vi "Set Start Parameter.vi"(8 "error in (no error)":errorcluster, 10 "Start Parameter":T2={"Windows Titel"="", "Start WorkDir"=path "C:/Users/user/Desktop/test/WorkDir", "Camera ConfigDir"=path "C:/Users/user/Desktop/test/ConfigDir", "Camera"="TestCam"}, 11 "HIJ 4 Aligment Cams Launcher in":refnum<class "HIJ 3 Aligment Cams Launcher.lvclass">) -> (0 "error out":errorcluster, 3 "HIJ 4 Aligment Cams Launcher out":refnum<class "HIJ 3 Aligment Cams Launcher.lvclass">)   [LabVIEW 2014, in "HIJ 3 Alignment Cams App.lvlib" / "HIJ 3 Aligment Cams Launcher.lvclass"]
uses:
  HIJ 3 Aligment Cams Launcher.lvclass
  <vilib>/userdefined/High Color/IMAQdx.ctl
  HIJ 3 Alignment Cams App/HIJ 3 Alignment Cams App.lvclass
  HIJ Vision Launcher/HIJ Vision Launcher/HIJ Vision Launcher.lvclass/HIJ Vision Launcher.ctl
  HIJ 3 Alignment Cams App/HIJ 3 Alignment Cams App.lvclass/HIJ 3 Alignment Cams App.ctl
  HIJ Vision Launcher/HIJ Vision Launcher/Read HIJ Vision Camera App.vi
  HIJ 3 Alignment Cams App/Write Start WorkDir.vi
  HIJ 3 Alignment Cams App/Write Start ConfigDir.vi
  HIJ 3 Alignment Cams App/Write Start Camera 1.vi
  HIJ Vision Launcher/HIJ Vision Launcher/Write HIJ Vision Camera App.vi
  Shared Code/Viewable Actor/ViewableActor/ViewableActor.lvclass
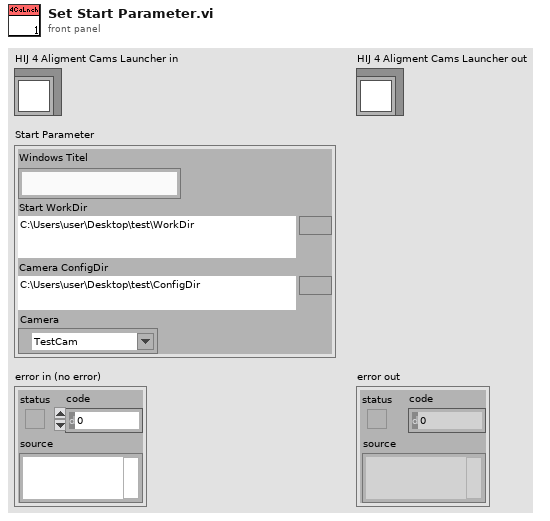
[diagram p1: front panel]
types:
  T1 = typedef "IMAQdx.ctl" = refnum<k21>
  T2 = cluster{"Windows Titel":string, "Start WorkDir":path, "Camera ConfigDir":path, "Camera":T1}
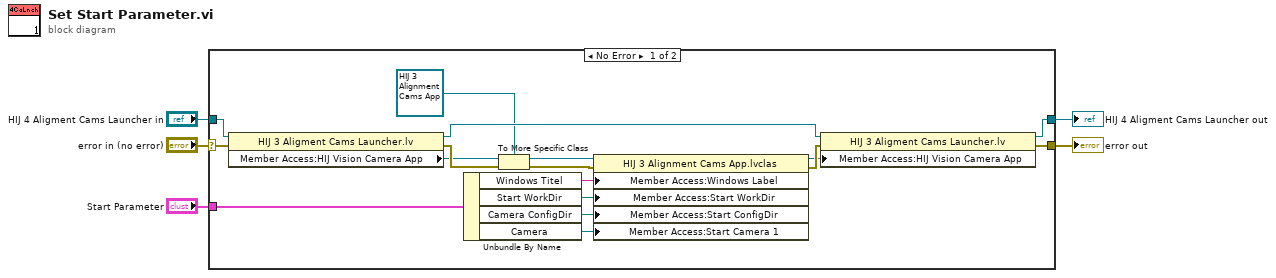
[diagram p0: block diagram]
diagram:
  n1 = case shown="No Error" "error in (no error)" {
    selector: "error in (no error)" -> [w12 w24]
    tunnel: [w9 w24] -> w2
    tunnel: [w14 w23] -> w1
    tunnel: "HIJ 4 Aligment Cams Launcher in" -> [w15 w23]
    tunnel: "Start Parameter" -> [w19 _]
    frame No Error {
      n2 = property class="HIJ 3 Aligment Cams Launcher.lv"(reference=w15, error in=w12) -> (reference out=w13:refnum<class "HIJ 3 Aligment Cams Launcher.lvclass">, error out=w11:errorcluster, "Member Access:HIJ Vision Camera App"=w7:refnum<class "ViewableActor.lvclass">)
      n3 = Unbundle By Name(w19) -> ("Windows Titel"=w22:string, "Start WorkDir"=w18:path, "Camera ConfigDir"=w17:path, "Camera"=w16:T1)
      n4 = To More Specific Class(target class=refnum<class "HIJ 3 Alignment Cams App.lvclass"> refnum ("HIJ 4 Alignment Cams App.lvlib:HIJ 4 Alignment Cams App.lvclass"), reference=w7, error in=w11) -> (specific class reference=w21:refnum<class "HIJ 3 Alignment Cams App.lvclass">, error out=w20:errorcluster)
      n5 = property class="HIJ 3 Alignment Cams App.lvclas"(reference=w21, error in=w20, "Member Access:Windows Label"=w22, "Member Access:Start WorkDir"=w18, "Member Access:Start ConfigDir"=w17, "Member Access:Start Camera 1"=w16) -> (reference out=w6:refnum<class "HIJ 3 Alignment Cams App.lvclass">, error out=w10:errorcluster)
      n6 = property class="HIJ 3 Aligment Cams Launcher.lv"(reference=w13, error in=w10, "Member Access:HIJ Vision Camera App"=w6) -> (reference out=w14:refnum<class "HIJ 3 Aligment Cams Launcher.lvclass">, error out=w9:errorcluster)
    }
    frame Error {
    }
  }
  "error out" <- w2
  "HIJ 4 Aligment Cams Launcher out" <- w1
